vi "Get streamai_signalConfig.vi"(8 "error in (no error)":errorcluster, 11 "gRPCid":T1) -> (0 "error out":errorcluster, 2 "package_templatemessage":T2, 3 "gRPCid out":T1)   [LabVIEW 2023, in "Generated_server.lvlib"]
uses:
  Generated_server.lvlib
  streamai_signalConfig.ctl
  streamai_SignalType.ctl
  <vilib>/gRPC/LabVIEW gRPC Library/Shared/grpcId.ctl
  streamai_signalConfig_Flat.ctl
  2ed25e12-861d-4677-8ead-ace2906b2041.vi
  <vilib>/gRPC/LabVIEW gRPC Library/Shared/TranslateGrpcError.vi
  <vilib>/gRPC/LabVIEW gRPC Library/Server API/Server/Get Server DLL Path.vi
  <vilib>/Utility/error.llb/Error Cluster From Error Code.vi
  <vilib>/gRPC/LabVIEW gRPC Library/grpc-lvsupport-release.lvlib
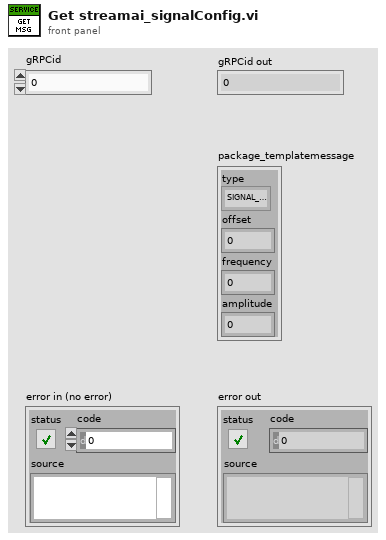
[diagram p1: front panel]
types:
  T1 = typedef "grpc-lvsupport-release.lvlib/grpcId.ctl" = u64
  T2 = typedef "Generated_server.lvlib/streamai_signalConfig.ctl" = cluster{"type":T3, "offset":dbl, "frequency":dbl, "amplitude":dbl}
  T3 = typedef "Generated_server.lvlib/streamai_SignalType.ctl" = enum32{"SIGNAL_SINE", "SIGNAL_SQUARE"}
  T4 = typedef "Generated_server.lvlib/streamai_signalConfig_Flat.ctl" = cluster{"type":T3, "offset":dbl, "frequency":dbl, "amplitude":dbl}
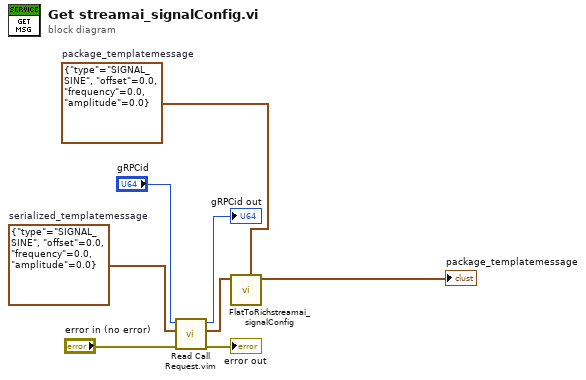
[diagram p0: block diagram]
diagram:
  w6 = T4 {"type"=enum."SIGNAL_SINE", "offset"=0.0, "frequency"=0.0, "amplitude"=0.0}  # serialized_templatemessage
  w5 = T2 {"type"=enum."SIGNAL_SINE", "offset"=0.0, "frequency"=0.0, "amplitude"=0.0}  # package_templatemessage
  n1 = call "Read Call Request.vim"("error in"="error in (no error)", "Request Type"=w6, "gRPCid in"="gRPCid") -> ("error out"=→"error out":errorcluster, "Request Data"=w4:T4, "gRPCid out"=→"gRPCid out":T1)  [unwired: 6 in]
  n2 = call "FlatToRichstreamai_signalConfig.vi"("OutputClusterType"=w5, "InputCluster"=w4) -> ("OutputCluster"=→"package_templatemessage":T2)  [unwired: 9 in]
